vi "Index.vi"(8 "error in (no error)":errorcluster, 10 "Index":i32, 11 "Generic Data in":refnum<class "Generic Data.lvclass">) -> (0 "error out":errorcluster, 3 "Indexed element":refnum<class "Generic Data.lvclass">)   [LabVIEW 2020, in "Data.lvlib" / "Generic Data.lvclass"]
doc: "Index an element from 'Generic Data in'.\nThe default implementation returns 'Generic Data in' as the 'Indexed element'."
uses:
  Generic Data.lvclass
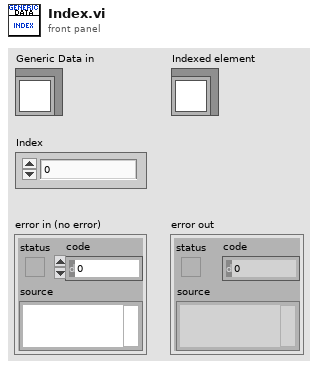
[diagram p1: front panel]
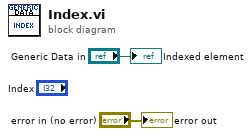
[diagram p0: block diagram]
diagram:
  "error out" <- "error in (no error)"
  "Indexed element" <- "Generic Data in"
